vi "Get IO Variable Contents.vi"(8 "error in (no error)":errorcluster, 11 "AllVariables[]":refnum<k21>[](array[refnum])) -> (0 "error out":errorcluster, 3 "All Variables Contents":T1[](array[typedef]))   [LabVIEW 2019, in "SEECD System Explorer.lvlib"]
uses:
  SEECD System Explorer.lvlib
  Type Defs/IOV Container Contents.ctl
  <resource>/objmgr/ni.var.rc
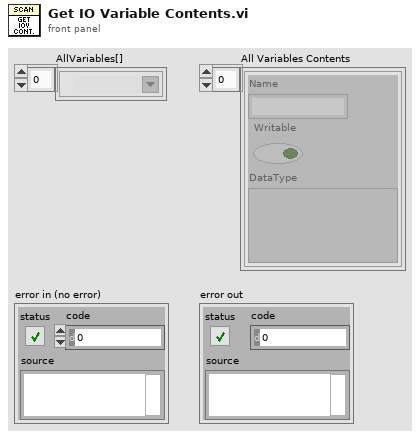
[diagram p1: front panel]
types:
  T1 = typedef "SEECD System Explorer.lvlib/IOV Container Contents.ctl" = cluster{"Name":string, "Writable":bool, "DataType":variant}
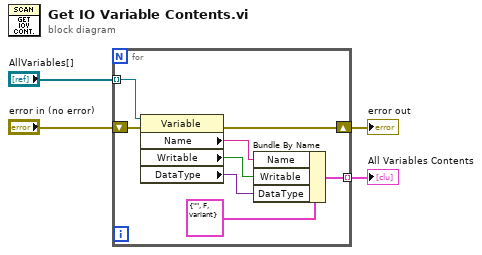
[diagram p0: block diagram]
diagram:
  n1 = for {
    tunnel: "AllVariables[]" -> [w12] mode=indexing
    shift-right: [w10] -> w4
    shift-left: "error in (no error)" -> [w11]
    tunnel: [w5] -> w3 mode=indexing
    n2 = property class="Variable"(reference=w12, error in=w11) -> (error out=w10:errorcluster, "Name"=w8:string, "Writable"=w7:bool, "DataType"=w6:variant)  [unwired: 1 out]
    n3 = Bundle By Name(cluster=T1 {"Name"="", "Writable"=FALSE, "DataType"=variant} ("IO Variable Container Contents"), "Name"=w8, "Writable"=w7, "DataType"=w6) -> (w5:T1)
  }
  "error out" <- w4
  "All Variables Contents" <- w3
